vi "Initialize Transfers.vi"(8 "error in (no error)":errorcluster, 11 "transfer configurations":T1[](array[typedef]) {"channels"."string offset" format="%d bytes"}) -> (0 "error out":errorcluster, 3 "transfers":T6[](array[typedef]))   [LabVIEW 2017, in "PXImc.lvlib" / "PXImc Transceiver.lvclass"]
uses:
  PXImc Transceiver.lvclass
  PXImc Transfer Data.ctl
  Builds/Data Sharing Framework/Current/Core/DSF Core.lvlibp/Typedefs/DSF Engine Transfer Configuration.ctl
  Builds/Data Sharing Framework/Current/Core/DSF Core.lvlibp/Typedefs/DSF Byte Order.ctl
  Builds/Data Sharing Framework/Current/Core/DSF Core.lvlibp/Typedefs/DSF Settings Info.ctl
  Builds/Data Sharing Framework/Current/Core/DSF Core.lvlibp/Typedefs/DSF Engine Channel Configuration.ctl
  Builds/Data Sharing Framework/Current/Core/DSF Core.lvlibp/Typedefs/DSF Data Type.ctl
  Builds/Data Sharing Framework/Current/Core/DSF Core.lvlibp/Classes/Configuration/Configuration Session.lvclass
  Builds/Data Sharing Framework/Current/Core/DSF Core.lvlibp
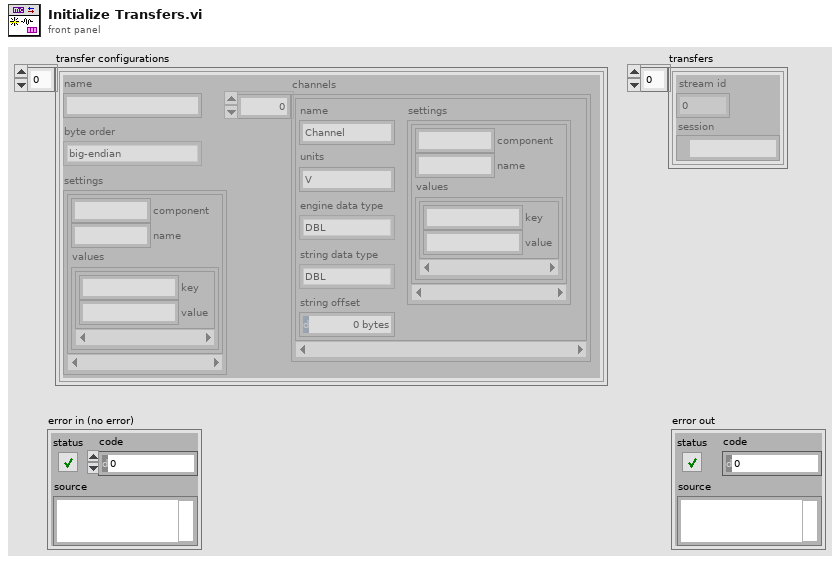
[diagram p1: front panel]
types:
  T1 = typedef "DSF Core.lvlibp/DSF Engine Transfer Configuration.ctl" = cluster{"name":string, "byte order":T2, "settings":T3, "channels":T4[]}
  T2 = typedef "DSF Core.lvlibp/DSF Byte Order.ctl" = enum8{"big-endian", "little-endian"}
  T3 = typedef "DSF Core.lvlibp/DSF Settings Info.ctl" = cluster{"component":string, "name":string, "values":cluster{"key":string, "value":string}[]}[]
  T4 = typedef "DSF Core.lvlibp/DSF Engine Channel Configuration.ctl" = cluster{"string offset":u64, "name":string, "units":string, "engine data type":T5, "string data type":T5, "settings":T3}
  T5 = typedef "DSF Core.lvlibp/DSF Data Type.ctl" = enum8{"Bool", "SGL", "DBL", "I8", "I16", "I32", "I64", "U8", "U16", "U32", "U64"}
  T6 = typedef "PXImc.lvlib/PXImc Transceiver.lvclass/PXImc Transfer Data.ctl" = cluster{"stream id":u16, "session":refnum<k21>}
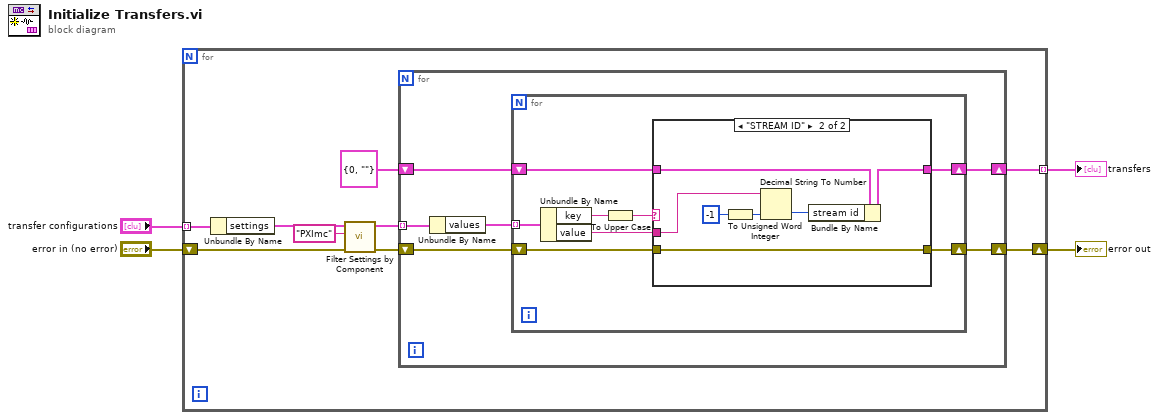
[diagram p0: block diagram]
diagram:
  n1 = for {
    tunnel: "transfer configurations" -> [w13] mode=indexing
    tunnel: [w7] -> w2 mode=indexing
    shift-right: [w6] -> w3
    shift-left: "error in (no error)" -> [w5]
    n2 = Unbundle By Name(w13) -> ("settings"=w12:T3)
    n3 = call "Filter Settings by Component.vi"("error in (no error)"=w5, "component"="PXImc", "settings"=w12) -> ("error out"=w9:errorcluster, "filtered settings"=w10:T3)  [unwired: 7 in]
    n4 = for {
      tunnel: w10 -> [w19] mode=indexing
      shift-right: [w14] -> w6
      shift-left: w9 -> [w17]
      shift-right: [w15] -> w7
      shift-left: T6 {"stream id"=0, "session"=""} ("PXImc Transfer") -> [w16]
      n5 = Unbundle By Name(w19) -> ("values"=w18:cluster{"key":string, "value":string}[])
      n6 = for {
        tunnel: w18 -> [w27] mode=indexing
        shift-right: [w20] -> w14
        shift-left: w17 -> [w23]
        shift-right: [w21] -> w15
        shift-left: w16 -> [w22]
        n7 = Unbundle By Name(w27) -> ("key"=w26:string, "value"=w24:string)
        n8 = To Upper Case(1:w26) -> (0:w25:string)
        n9 = case shown="\"STREAM ID\"" w25 {
          tunnel: w24 -> [_ w36]
          tunnel: w23 -> [w28 w30]
          tunnel: w22 -> [w29 w32]
          tunnel: [w29 w31] -> w21
          tunnel: [w28 w30] -> w20
          frame Default {
            # "Unknown setting"
          }
          frame "STREAM ID" {
            n10 = To Unsigned Word Integer(number=i16 -1 ("default (0 I32)")) -> (unsigned 16bit integer=w34:u16)
            n11 = Decimal String To Number(string=w36, default (0L)=w34) -> (number=w33:u16)  [unwired: 1 in, 1 out]
            n12 = Bundle By Name(cluster=w32, "stream id"=w33) -> (w31:T6)
          }
        }
      }
    }
  }
  "error out" <- w3
  "transfers" <- w2
